vi "EncodeUInt32.vi"(1 "Data In":u32[](array[numeric])) -> (0 "Data Out":u8[](array[numeric]))   [LabVIEW 2015, in "navX Library v1 (deprecated).lvlib"]
uses:
  navX Library v1 (deprecated).lvlib
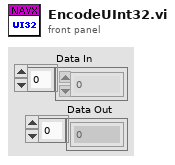
[diagram p1: front panel]
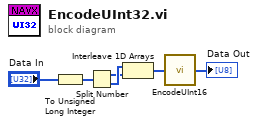
[diagram p0: block diagram]
diagram:
  n1 = To Unsigned Long Integer(number="Data In") -> (unsigned 32bit integer=w1:u32[])
  n2 = Split Number(x=w1) -> (hi(x)=w3:u16[], lo(x)=w4:u16[])
  n3 = Interleave 1D Arrays(w4, w3) -> (w2:u16[])
  n4 = call "EncodeUInt16.vi"("Data In"=w2) -> ("Data Out"=→"Data Out":u8[])
